vi "Get Error Description from Error No.vi"(11 "Error Number":T1 items=["ERR_NOERROR"=0, "ERR_ACCESS_OUTPUTFOLDER"=1, "ERR_INVALID_LIBRARYNAME"=2, "ERR_CREATE_VIWRAPPER"=3, "ERR_UNKNOWN"=201, "ERR_BAD_ARGUMENT"=202, "ERR_URL_NOTFOUND_BADWSDL"=203, "ERR_BADLYFORMATTEDURL"=204, "ERR_BADHOSTNAME"=205, "ERR_BADDIRECTORY"=206, "ERR_UNAUTHORIZEDACCESS"=207, "ERR_CREATELIBRARY"=208, "ERR_COMPILEERROR"=209]) -> (1 "Error Description":string, 2 "Error Title":string, 3 "Found?":bool)   [LabVIEW 2017, in "WebServiceImporter.lvlib" / "Error Handling.lvlib"]
uses:
  <vilib>/Platform/WebService/Error Handling/Error Handling.lvlib
  <vilib>/Platform/WebService/Error Handling/Error/Error Number.ctl
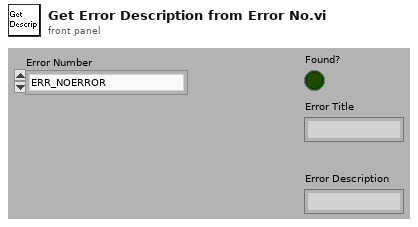
[diagram p1: front panel]
types:
  T1 = typedef "WebServiceImporter.lvlib/Error Handling.lvlib/Error Number.ctl" = u16
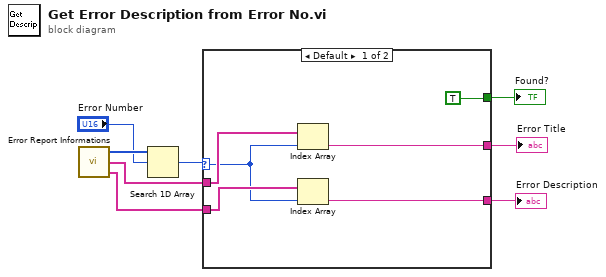
[diagram p0: block diagram]
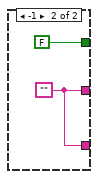
[diagram p2: hidden frame]
diagram:
  n1 = call <vilib>:"Error Report Informations.vi"() -> ("Error Descriptions Out"=w3:string[], "Error Titles Out"=w4:string[], "Error Numbers Out"=w8:T1[])
  n2 = Search 1D Array(1D array=w8, element="Error Number") -> (index of element=w6:i32)  [unwired: 1 in]
  n3 = case shown="Default" w6 {
    selector: w6 -> [w11 _]
    tunnel: [TRUE FALSE] -> w5
    tunnel: w4 -> [w13 _]
    tunnel: w3 -> [w12 _]
    tunnel: [w10 w15] -> w1
    tunnel: [w9 w15] -> w2
    frame Default {
      n4 = Index Array(array=w13, index=w11) -> (element=w10:string)
      n5 = Index Array(array=w12, index=w11) -> (element=w9:string)
    }
    frame -1 {
      w15 = ""
    }
  }
  "Error Title" <- w1
  "Found?" <- w5
  "Error Description" <- w2
